vi "Sub_VI_Aleatorio-Furo.vi"(9 "Altura do Tanque":dbl, 10 "Altura do Furo":dbl, 11 "Havia Furo?":bool) -> (2 "Boolean out":bool, 3 "Altura do Furo":dbl)   [LabVIEW 2019]
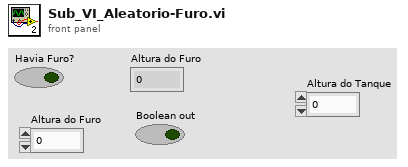
[diagram p1: front panel]
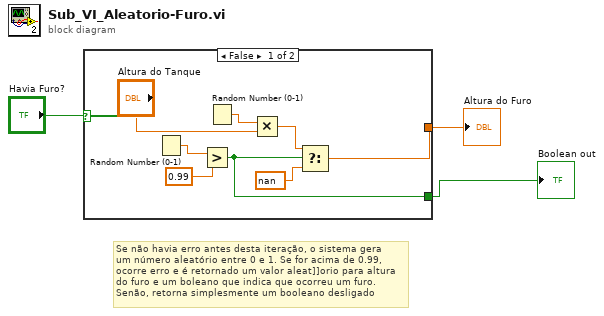
[diagram p0: block diagram]
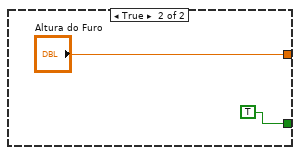
[diagram p2: hidden frame]
diagram:
  # "Se não havia erro antes desta iteração, o sistema gera\num número aleatório entre 0 e 1. Se for acima de 0.99,\nocorre erro e é retornado um valor aleat]]orio para altura\ndo furo e um boleano que indica que ocorreu um furo.\nSenão, retorna simplesmente um booleano desligado"
  n1 = case shown="False" "Havia Furo?" {
    tunnel: [w9 "Altura do Furo"] -> w2
    tunnel: [w5 TRUE] -> w1
    frame False {
      n2 = Random Number (0-1)() -> (number: 0 to 1=w10:dbl)
      n3 = Greater?(x=w10, y=0.99) -> (0:w5:bool)
      n4 = Random Number (0-1)() -> (number: 0 to 1=w8:dbl)
      n5 = Multiply(x=w8, y="Altura do Tanque") -> (x*y=w7:dbl)
      n6 = Select(t=w7, s=w5, f=nan) -> (s? t:f=w9:dbl)
    }
    frame True {
    }
  }
  "Boolean out" <- w1
  "Altura do Furo" <- w2
